vi "1A Helper - Generate RegEx.vi"(1 "# Datums":i32) -> (0 "RegEx":string)   [LabVIEW 2011]
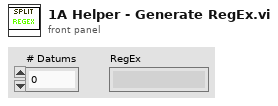
[diagram p1: front panel]
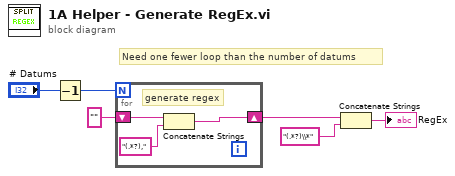
[diagram p0: block diagram]
diagram:
  # "Need one fewer loop than the number of datums"
  n1 = Decrement(x="# Datums") -> (x-1=w4:i32)
  n2 = for {
    N: w4 -> [_]
    shift-right: [w7] -> w3
    shift-left: "" -> [w9]
    # "generate regex"
    n3 = Concatenate Strings(w9, "(.*?),") -> (w7:string)
  }
  n4 = Concatenate Strings(w3, "(.*?)\\*") -> (→"RegEx":string)
